vi "milisecondsToTime.vi"(11 "Time input":dbl) -> (3 "Time Stamp":string)   [LabVIEW 2021]
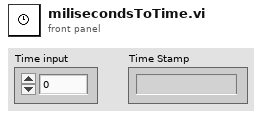
[diagram p1: front panel]
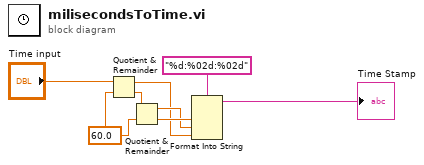
[diagram p0: block diagram]
diagram:
  w8 = 60.0 ("y")
  n1 = Quotient & Remainder(x="Time input", y=w8) -> (x-y*floor(x/y)=w2:dbl, floor(x/y)=w1:dbl)
  n2 = Quotient & Remainder(x=w1, y=w8) -> (x-y*floor(x/y)=w3:dbl, floor(x/y)=w4:dbl)
  n3 = Format Into String(format string="%d:%02d:%02d", w4, w3, w2) -> (resulting string=→"Time Stamp":string)  [unwired: 2 in, 1 out]
